vi "Technosoft_init.vi"(8 "error in (no error)":errorcluster, 11 "VISA resource name":refnum<visa-resource-name>) -> (0 "error out":errorcluster, 3 "VISA resource name out":refnum<visa-resource-name>, 5 "Try baud":i32)   [LabVIEW 2011]
uses:
  <vilib>/Instr/_visa.llb/VISA Flush IO Buffer Mask.ctl
panel:
  out "test loop":i32
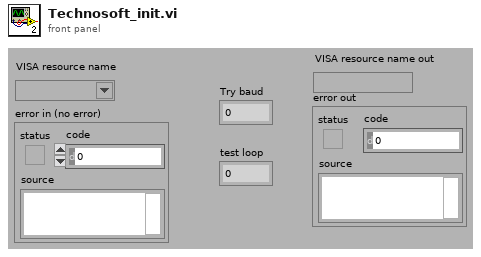
[diagram p1: front panel]
types:
  T1 = typedef "VISA Flush IO Buffer Mask.ctl" = u16
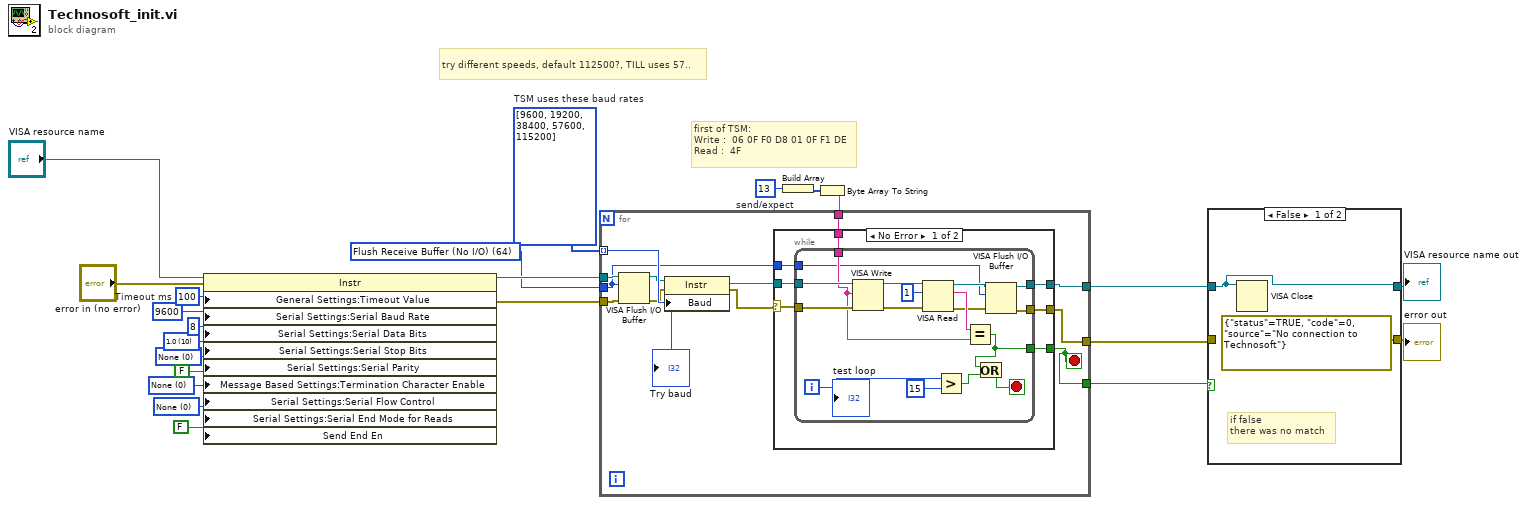
[diagram p0: block diagram]
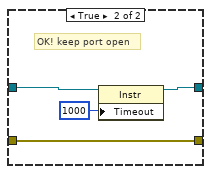
[diagram p2: hidden frame]
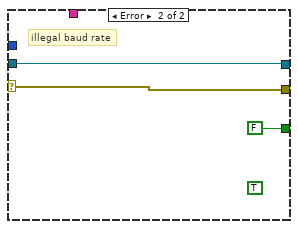
[diagram p3: hidden frame]
diagram:
  w7 = T1 64 items=["Flush Receive Buffer"=16, "Write Transmit Buffer to Device"=32, "Flush Receive Buffer (No I/O)"=64, "Flush Transmit Buffer"=128] ("Mask")
  w15 = u8 13  # send/expect
  w17 = u32 100  # Timeout ms
  w19 = u16 10 items=["1.0"=10, "1.5"=15, "2.0"=20] ("Serial Settings:Stop Bits")
  w20 = u16 0 items=["None", "Odd", "Even", "Mark", "Space"] ("Serial Settings:Parity")
  w21 = u16 0 items=["None", "Last Bit", "TermChar"] ("Serial Settings:End Mode for Reads")
  w22 = u16 0 items=["None", "XON/XOFF", "RTS/CTS", "XON/XOFF & RTS/CTS", "DTR/DSR", "XON/XOFF & DTR/DSR"] ("Serial Settings:Flow Control")
  w12 = i32[] [9600, 19200, 38400, 57600, 115200]  # TSM uses these baud rates
  # "try different speeds, default 112500?, TILL uses 57.."
  # "first of TSM:\nWrite :  06 0F F0 D8 01 0F F1 DE\nRead :  4F"
  n1 = property class="Instr"(reference="VISA resource name", error in="error in (no error)", "General Settings:Timeout Value"=w17, "Serial Settings:Serial Baud Rate"=u32 9600 ("Serial Settings:Baud Rate"), "Serial Settings:Serial Data Bits"=u16 8 ("Serial Settings:Data Bits"), "Serial Settings:Serial Stop Bits"=w19, "Serial Settings:Serial Parity"=w20, "Message Based Settings:Termination Character Enable"=FALSE, "Serial Settings:Serial Flow Control"=w22, "Serial Settings:Serial End Mode for Reads"=w21, "Send End En"=FALSE ("Message Based Settings:Send End Enable")) -> (reference out=w9:refnum<visa-resource-name>, error out=w8:errorcluster)
  n2 = Build Array(w15) -> (w10:u8[])
  n3 = Byte Array To String(unsigned byte array=w10) -> (string=w11:string)
  n4 = for {
    tunnel: w12 -> [w34] mode=indexing
    tunnel: [w33] -> w4
    tunnel: [w31] -> w5
    tunnel: w11 -> [w30]
    tunnel: w9 -> [w28]
    tunnel: w8 -> [w27]
    tunnel: w7 -> [w25]
    tunnel: [w24] -> w6
    stop <- w24 stop-if-true
    n5 = VISA Flush I/O Buffer(VISA resource name=w28, mask (16)=w25, error in (no error)=w27) -> (VISA resource name out=w29:refnum<visa-resource-name>, error out=w26:errorcluster)
    n6 = property class="Instr"(reference=w29, error in=w26, "Baud"=w34) -> (reference out=w35:refnum<visa-resource-name>, error out=w32:errorcluster)
    n7 = case shown="No Error" w32 {
      selector: w32 -> [w39 w61]
      tunnel: w35 -> [w42 w62]
      tunnel: [w41 FALSE] -> w24
      tunnel: [w40 w62] -> w33
      tunnel: [w38 w61] -> w31
      tunnel: w30 -> [w37 _]
      tunnel: w25 -> [w36 _]
      frame No Error {
        n8 = while {
          tunnel: w42 -> [w59]
          tunnel: w39 -> [w58]
          tunnel: [w47] -> w40
          tunnel: [w52] -> w41
          tunnel: [w45] -> w38
          tunnel: w37 -> [w49]
          tunnel: w36 -> [w44]
          i -> [w51]
          stop <- w53 stop-if-true
          n9 = VISA Write(VISA resource name=w59, write buffer=w49, error in (no error)=w58) -> (VISA resource name out=w57:refnum<visa-resource-name>, error out=w55:errorcluster)  [unwired: 1 out]
          n10 = VISA Read(VISA resource name=w57, byte count=u32 1, error in (no error)=w55) -> (VISA resource name out=w48:refnum<visa-resource-name>, read buffer=w50:string, error out=w46:errorcluster)  [unwired: 1 out]
          n11 = Greater?(x=w51, y=15) -> (0:w43:bool)
          n12 = Equal?(x=w50, y=w49) -> (x = y?=w52:bool)
          n13 = Or(x=w52, y=w43) -> (x .or. y?=w53:bool)
          n14 = VISA Flush I/O Buffer(VISA resource name=w48, mask (16)=w44, error in (no error)=w46) -> (VISA resource name out=w47:refnum<visa-resource-name>, error out=w45:errorcluster)
          "test loop" <- w51
        }
      }
      frame Error {
        (unwired) TRUE
        # "illegal baud rate"
      }
    }
    "Try baud" <- w34
  }
  n15 = case shown="False" w6 {
    tunnel: w5 -> [_ w67]
    tunnel: w4 -> [w64 w68]
    tunnel: [w64 w66] -> w3
    tunnel: [errorcluster {"status"=TRUE, "code"=0, "source"="No connection to Technosoft"} ("error IO") w67] -> w2
    frame False {
      # "if false \nthere was no match"
      n16 = VISA Close(VISA resource name=w64) -> ()  [unwired: 1 in, 1 out]
    }
    frame True {
      # "OK! keep port open"
      n17 = property class="Instr"(reference=w68, "Timeout"=u32 1000 ("General Settings:Timeout Value")) -> (reference out=w66:refnum<visa-resource-name>)  [unwired: 1 in, 1 out]
    }
  }
  "VISA resource name out" <- w3
  "error out" <- w2
